vi "Teleop (Christian Colglazier's conflicted copy 2013-02-10).vi"(10 "Match Info":T1={"Autonomous Elapsed Seconds"=0.0, "TeleOp Elapsed Seconds"=0.0, "Disabled Elapsed Seconds"=0.0, "Visited Autonomous"=FALSE, "Visited TeleOp"=FALSE, "Visited Disabled"=FALSE, "Autonomous Settings"={"Autonomous Style"=enum."Independent", "VI Refnum"=refnum}}, 11 "Call Context":T2) -> ()   [LabVIEW 2012]
doc: "This VI is called for each TeleOp packet received from the DS where the robot is not disabled. It is often used to read from the joysticks and update I/O or to update setpoints for timed control loops. It should complete and return within 20 milliseconds or it may miss DS packets."
uses:
  <vilib>/Rock Robotics/WPI/DriverStation/WPI_DriverStationDerivedRobotMode.ctl
  <vilib>/Rock Robotics/WPI/DriverStation/WPI_DriverStationMatch Info.ctl
  Robot Global Data.vi
  <vilib>/Rock Robotics/WPI/Joystick/WPI_JoystickGetSetRefNum.vi
  <vilib>/Rock Robotics/WPI/RobotDrive/WPI_RobotDriveGetSetRefNum.vi
panel:
  out "Numeric 1":dbl(slide) scale=0.0..100.0
  out "Boolean 2":bool
  out "Boolean 1":bool
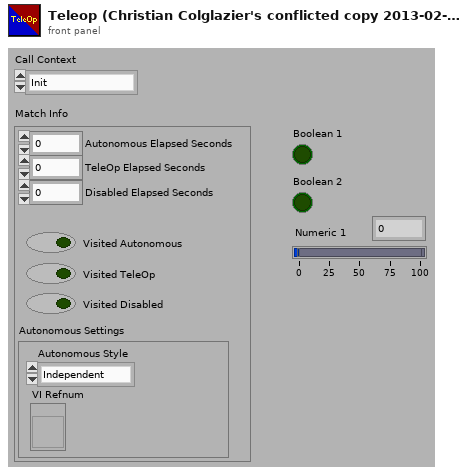
[diagram p1: front panel]
types:
  T1 = typedef "WPI_DriverStationMatch Info.ctl" = cluster{"Autonomous Elapsed Seconds":dbl, "TeleOp Elapsed Seconds":dbl, "Disabled Elapsed Seconds":dbl, "Visited Autonomous":bool, "Visited TeleOp":bool, "Visited Disabled":bool, "Autonomous Settings":cluster{"Autonomous Style":enum16{"Iterative", "Independent"}, "VI Refnum":refnum<vi>}}
  T2 = typedef "WPI_DriverStationDerivedRobotMode.ctl" = enum16{"Init", "Execute", "Stop"}
  T3 = typedef "WPI_RobotDriveDevRef.ctl" = cluster{"DevStatus":errorcluster, "Motors[]":T4[], "Square Inputs":bool, "Max Output":dbl, "Isochronous":bool}
  T4 = typedef "WPI_MotorControlDeviceRef.ctl" = cluster{"DeviceStatus":errorcluster, "Type":enum16{"PWM", "CAN"}, "PWM":cluster{"Digital Module":T5, "PWM Channel":T6, "DeadBand":T7}, "CAN":cluster{"Device Number":u8, "Control Mode":T8, "Semaphore":T9, "Max Vout":dbl}, "Invert":bool, "TransformRef":T10, "InvTransformRef":T10}
  T5 = typedef "FPGA_TypedefDigitalModule.ctl" = enum16{"Digital Module 1", "Digital Module 2"}
  T6 = typedef "FPGA_DIOPWMChannel.ctl" = enum8{"PWM 1", "PWM 2", "PWM 3", "PWM 4", "PWM 5", "PWM 6", "PWM 7", "PWM 8", "PWM 9", "PWM 10", "Invalid"}
  T7 = typedef "WPI_PWMDeadband.ctl" = cluster{"Name":string, "maxPositivePwm":i32, "minPositivePwm":i32, "centerPwm":i32, "maxNegativePwm":i32, "minNegativePwm":i32, "angularRange":u16}
  T8 = typedef "WPI_CANJaguar_ControlMode.ctl" = enum8{"Percent VBus", "Current", "Speed", "Position", "Voltage"}
  T9 = typedef "Semaphore RefNum" = refnum<k1>
  T10 = typedef "WPI_PWMTransform_ConPane.ctl" = refnum<vi>
  T11 = typedef "WPI_JoystickDevRef.ctl" = cluster{"Device":T12}
  T12 = typedef "WPI_JoystickDeviceEnum.ctl" = enum16{"USB 1", "USB 2", "USB 3", "USB 4", "Kinect 1", "Kinect 2"}
  T13 = typedef "WPI_JoystickButtonState.ctl" = cluster{"Button 1":bool, "Button 2":bool, "Button 3":bool, "Button 4":bool, "Button 5":bool, "Button 6":bool, "Button 7":bool, "Button 8":bool, "Button 9":bool, "Button 10":bool, "Button 11":bool, "Button 12":bool}
  T14 = cluster{"axis 1 (x)":dbl, "axis 2 (y)":dbl, "axis 3 (throttle)":dbl, "axis 4":dbl, "axis 5":dbl, "axis 6":dbl}
  T15 = typedef "WPI_AccelerometerDevRef.ctl" = cluster{"DevStatus":errorcluster, "Analog Module":T16, "Analog Channel":T17, "Scaling":T18}
  T16 = typedef "FPGA_TypedefAnalogModule.ctl" = enum16{"Analog Module 1", "Analog Module 2"}
  T17 = typedef "FPGA_AIChannel.ctl" = enum8{"AI 1", "AI 2", "AI 3", "AI 4", "AI 5", "AI 6", "AI 7", "AI 8", "Invalid"}
  T18 = typedef "WPI_AccelerometerScaling.ctl" = cluster{"Gain (VoltsPerG)":dbl, "Center Voltage":dbl}
  T19 = typedef "WPI_GyroDevRef.ctl" = cluster{"DevStatus":errorcluster, "Analog Module":T16, "Analog Channel":T17, "Offset":dbl, "Gain (VoltsPerDegree/Second)":dbl}
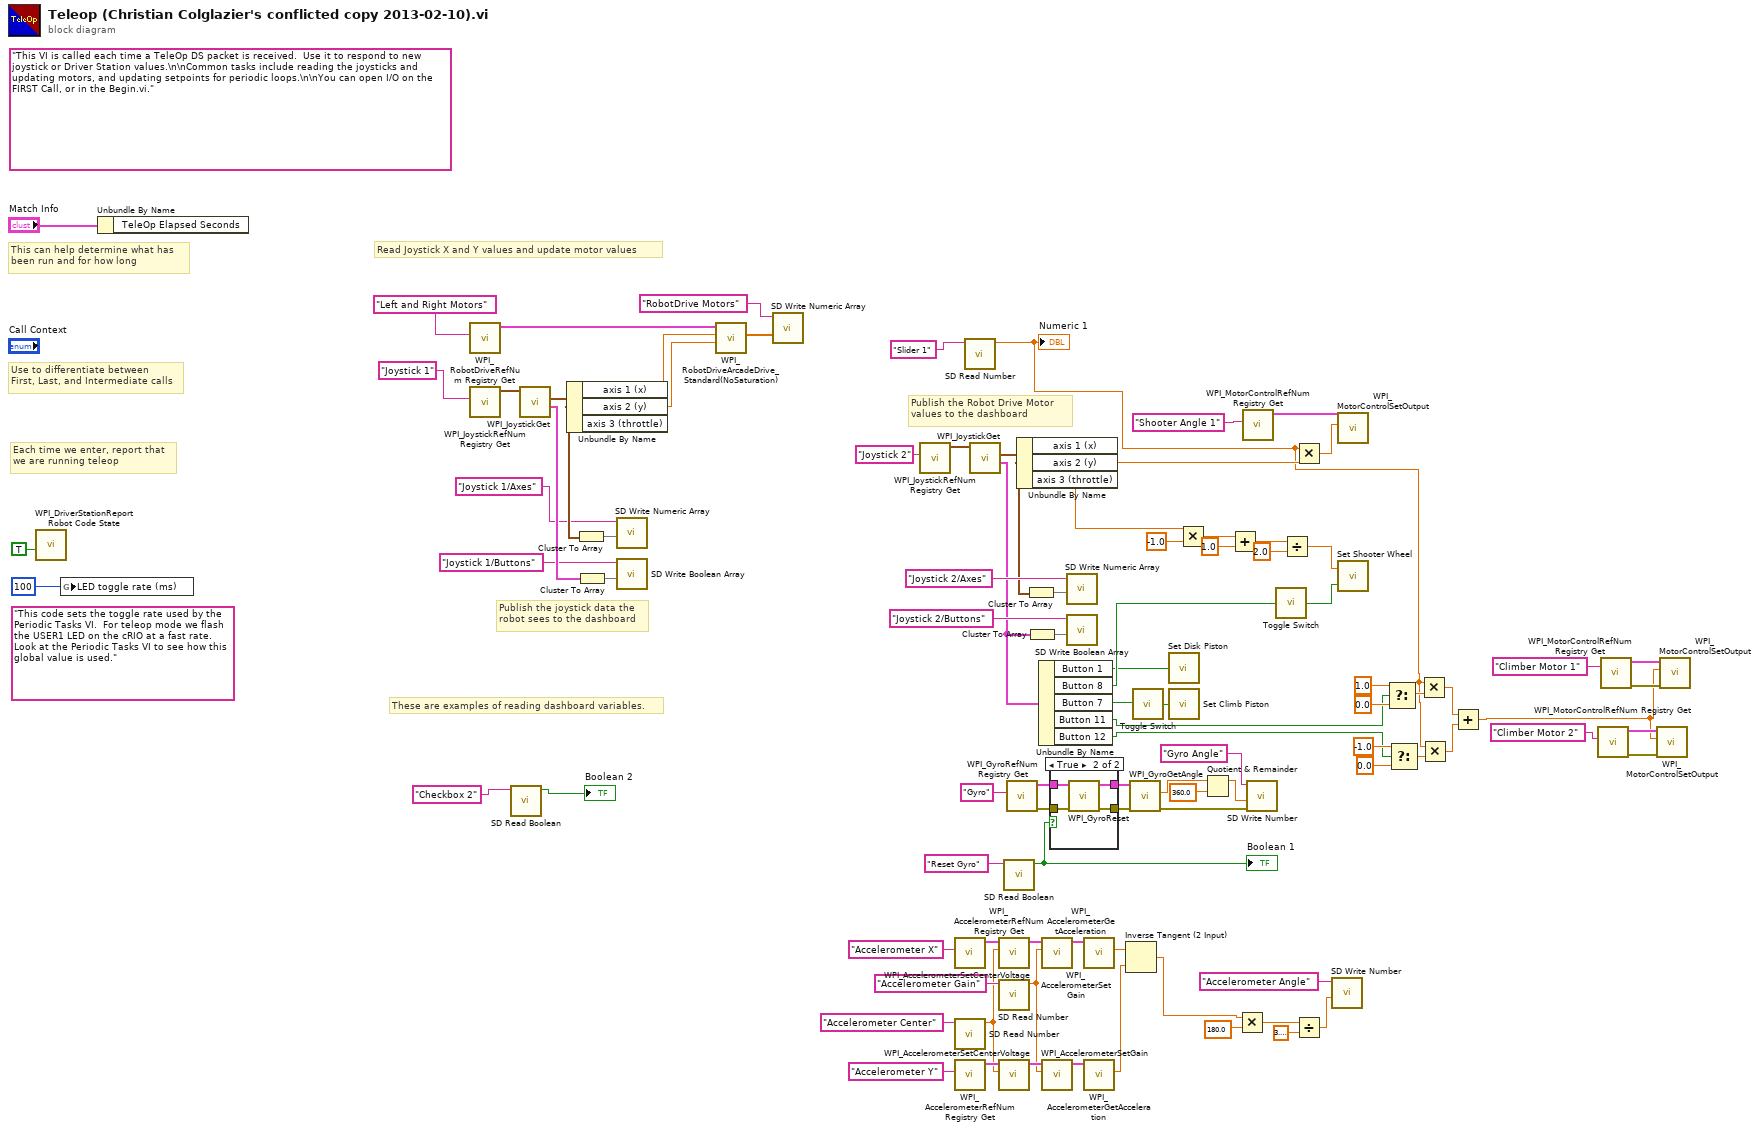
[diagram p0: block diagram]
diagram:
  (unwired) "This code sets the toggle rate used by the Periodic Tasks VI.  For teleop mode we flash the USER1 LED on the cRIO at a fast rate.  Look at the Periodic Tasks VI to see how this global value is used."
  (unwired) "This VI is called each time a TeleOp DS packet is received.  Use it to respond to new joystick or Driver Station values.\n\nCommon tasks include reading the joysticks and updating motors, and updating setpoints for periodic loops.\n\nYou can open I/O on the FIRST Call, or in the Begin.vi."
  # "These are examples of reading dashboard variables."
  # "Publish the Robot Drive Motor\nvalues to the dashboard"
  # "Publish the joystick data the\nrobot sees to the dashboard"
  # "Each time we enter, report that\nwe are running teleop"
  # "Use to differentiate between\nFirst, Last, and Intermediate calls"
  # "This can help determine what has\nbeen run and for how long"
  # "Read Joystick X and Y values and update motor values"
  n1 = call <vilib>:"WPI_DriverStationReport Robot Code State.vi"("TeleOp"=TRUE ("Autonomous")) -> ()  [unwired: 10 in, 1 out]
  n2 = global write "Robot Global Data.vi" "LED toggle rate (ms)"(u32 100 ("LED ms toggle rate")) -> ()
  n3 = Unbundle By Name("Match Info") -> ()  [unwired: 1 out]
  n4 = call <vilib>:"WPI_RobotDriveRefNum Registry Get.vi"("refnum name"="Left and Right Motors") -> ("RobotDriveDevRef"=w92:T3)  [unwired: 1 in, 9 out]
  n5 = call <vilib>:"WPI_JoystickRefNum Registry Get.vi"("refnum name"="Joystick 1") -> ("JoystickDevRef"=w88:T11)  [unwired: 1 in, 9 out]
  n6 = call <vilib>:"SD Read Boolean.vi"("Name"="Checkbox 2" ("refnum name")) -> ("Boolean"=→"Boolean 2":bool)  [unwired: 8 in, 2 out]
  n7 = call <vilib>:"WPI_JoystickGet.vi"("JoystickDevRef"=w88) -> ("Buttons"=w85:T13, "Axes"=w82:T14)  [unwired: 1 in, 4 out]
  n8 = Unbundle By Name(w82) -> ("axis 1 (x)"=w91:dbl, "axis 2 (y)"=w90:dbl)  [unwired: 1 out]
  n9 = Cluster To Array(cluster=w82) -> (array=w81:dbl[])
  n10 = Cluster To Array(cluster=w85) -> (array=w84:bool[])
  n11 = call <vilib>:"SD Write Numeric Array.vi"("Numeric Array"=w81, "Name"="Joystick 1/Axes") -> ()  [unwired: 8 in, 2 out]
  n12 = call <vilib>:"SD Write Boolean Array.vi"("Boolean Array"=w84, "Name"="Joystick 1/Buttons") -> ()  [unwired: 8 in, 2 out]
  n13 = call <vilib>:"WPI_RobotDriveArcadeDrive_Standard(NoSaturation).vi"("Y axis value"=w90, "X axis value"=w91, "RobotDriveDevRef"=w92) -> ("Motor Values"=w78:dbl[])  [unwired: 1 in, 7 out]
  n14 = call <vilib>:"SD Write Numeric Array.vi"("Numeric Array"=w78, "Name"="RobotDrive Motors") -> ()  [unwired: 8 in, 2 out]
  n15 = call <vilib>:"WPI_JoystickRefNum Registry Get.vi"("refnum name"="Joystick 2") -> ("JoystickDevRef"=w68:T11)  [unwired: 1 in, 9 out]
  n16 = call <vilib>:"WPI_AccelerometerRefNum Registry Get.vi"("refnum name"="Accelerometer X") -> ("AccelerometerDevRef"=w26:T15)  [unwired: 9 in, 1 out]
  n17 = call <vilib>:"SD Read Number.vi"("Name"="Accelerometer Center" ("refnum name")) -> ("Numeric"=w21:dbl)  [unwired: 8 in, 2 out]
  n18 = call <vilib>:"WPI_AccelerometerRefNum Registry Get.vi"("refnum name"="Accelerometer Y") -> ("AccelerometerDevRef"=w25:T15)  [unwired: 9 in, 1 out]
  n19 = call <vilib>:"SD Read Number.vi"("Name"="Slider 1" ("refnum name")) -> ("Numeric"=w6:dbl)  [unwired: 8 in, 2 out]
  "Numeric 1" <- w6
  n20 = call <vilib>:"WPI_JoystickGet.vi"("JoystickDevRef"=w68) -> ("Buttons"=w64:T13, "Axes"=w71:T14)  [unwired: 1 in, 4 out]
  n21 = call <vilib>:"WPI_AccelerometerSetCenterVoltage.vi"("Center Voltage"=w21, "AccelerometerDevRef"=w26) -> ("AccelerometerDevRef"=w36:T15)  [unwired: 1 in, 8 out]
  n22 = call <vilib>:"SD Read Number.vi"("Name"="Accelerometer Gain" ("refnum name")) -> ("Numeric"=w22:dbl)  [unwired: 8 in, 2 out]
  n23 = call <vilib>:"WPI_AccelerometerSetCenterVoltage.vi"("Center Voltage"=w21, "AccelerometerDevRef"=w25) -> ("AccelerometerDevRef"=w37:T15)  [unwired: 1 in, 8 out]
  n24 = call <vilib>:"SD Read Boolean.vi"("Name"="Reset Gyro" ("refnum name")) -> ("Boolean"=w46:bool)  [unwired: 8 in, 2 out]
  "Boolean 1" <- w46
  n25 = call <vilib>:"WPI_GyroRefNum Registry Get.vi"("refnum name"="Gyro") -> ("error out"=w41:errorcluster, "GyroDevRef"=w42:T19)  [unwired: 9 in]
  n26 = Unbundle By Name(w71) -> ("axis 2 (y)"=w63:dbl, "axis 3 (throttle)"=w57:dbl)  [unwired: 1 out]
  n27 = Cluster To Array(cluster=w71) -> (array=w72:dbl[])
  n28 = Cluster To Array(cluster=w64) -> (array=w69:bool[])
  n29 = Unbundle By Name(w64) -> ("Button 1"=w52:bool, "Button 8"=w61:bool, "Button 7"=w54:bool, "Button 11"=w14:bool, "Button 12"=w11:bool)
  n30 = call <vilib>:"WPI_AccelerometerSetGain.vi"("Gain (VoltsPerG)"=w22, "AccelerometerDevRef"=w36) -> ("AccelerometerDevRef"=w35:T15)  [unwired: 1 in, 8 out]
  n31 = call <vilib>:"WPI_AccelerometerSetGain.vi"("Gain (VoltsPerG)"=w22, "AccelerometerDevRef"=w37) -> ("AccelerometerDevRef"=w38:T15)  [unwired: 1 in, 8 out]
  n32 = case shown="True" w46 {
    tunnel: w42 -> [w96 w100]
    tunnel: w41 -> [w95 w99]
    tunnel: [w96 w98] -> w40
    tunnel: [w95 w97] -> w39
    frame False {
    }
    frame True {
      n33 = call <vilib>:"WPI_GyroReset.vi"("error in (no error)"=w99, "GyroDevRef"=w100) -> ("error out"=w97:errorcluster, "GyroDevRef"=w98:T19)  [unwired: 8 in]
    }
  }
  n34 = call <vilib>:"SD Write Numeric Array.vi"("Numeric Array"=w72, "Name"="Joystick 2/Axes") -> ()  [unwired: 8 in, 2 out]
  n35 = call <vilib>:"SD Write Boolean Array.vi"("Boolean Array"=w69, "Name"="Joystick 2/Buttons") -> ()  [unwired: 8 in, 2 out]
  n36 = call <vilib>:"WPI_AccelerometerGetAcceleration.vi"("AccelerometerDevRef"=w35) -> ("Acceleration"=w30:dbl)  [unwired: 1 in, 9 out]
  n37 = call <vilib>:"WPI_AccelerometerGetAcceleration.vi"("AccelerometerDevRef"=w38) -> ("Acceleration"=w29:dbl)  [unwired: 1 in, 9 out]
  n38 = Inverse Tangent (2 Input)(1:w29, 2:w30) -> (0:w31:dbl)
  n39 = call <vilib>:"WPI_GyroGetAngle.vi"("error in (no error)"=w39, "GyroDevRef"=w40) -> ("error out"=w48:errorcluster, "Angle"=w44:dbl)  [unwired: 6 in, 2 out]
  n40 = call "Toggle Switch.vi"("OK Button"=w54) -> ("Boolean 2"=w53:bool)
  n41 = call "Set Disk Piston.vi"("Boolean"=w52) -> ()
  n42 = call "Set Climb Piston.vi"("Boolean"=w53) -> ()
  n43 = Multiply(x=w57, y=-1.0) -> (x*y=w56:dbl)
  n44 = Quotient & Remainder(x=w44, y=360.0) -> (x-y*floor(x/y)=w43:dbl)  [unwired: 1 out]
  n45 = Add(x=w56, y=1.0) -> (x+y=w59:dbl)
  n46 = Multiply(x=w31, y=180.0) -> (x*y=w33:dbl)
  n47 = call <vilib>:"WPI_MotorControlRefNum Registry Get.vi"("refnum name"="Shooter Angle 1") -> ("MotorControlDevRef"=w65:T4)  [unwired: 9 in, 1 out]
  n48 = call <vilib>:"SD Write Number.vi"("error in"=w48, "Numeric"=w43, "Name"="Gyro Angle") -> ()  [unwired: 7 in, 2 out]
  n49 = call "Toggle Switch.vi"("OK Button"=w61) -> ("Boolean 2"=w51:bool)
  n50 = Divide(x=w59, y=2.0) -> (x/y=w50:dbl)
  n51 = Multiply(x=w6, y=w63) -> (x*y=w62:dbl)
  n52 = Divide(x=w33, y=3.141592653589793) -> (x/y=w20:dbl)
  n53 = call <vilib>:"SD Write Number.vi"("Numeric"=w20, "Name"="Accelerometer Angle") -> ()  [unwired: 8 in, 2 out]
  n54 = call <vilib>:"WPI_MotorControlSetOutput.vi"("Output"=w62, "MotorControlDevRef"=w65) -> ()  [unwired: 7 in, 3 out]
  n55 = call "Set Shooter Wheel.vi"("Reverse"=w51, "Motor Speed"=w50) -> ()  [unwired: 2 in]
  n56 = Select(t=1.0, s=w14, f=0.0) -> (s? t:f=w9:dbl)
  n57 = Select(t=-1.0, s=w11, f=0.0) -> (s? t:f=w10:dbl)
  n58 = Multiply(x=w6, y=w9) -> (x*y=w7:dbl)
  n59 = Multiply(x=w6, y=w10) -> (x*y=w8:dbl)
  n60 = Add(x=w7, y=w8) -> (x+y=w1:dbl)
  n61 = call <vilib>:"WPI_MotorControlRefNum Registry Get.vi"("refnum name"="Climber Motor 2") -> ("error out"=w3:errorcluster, "MotorControlDevRef"=w2:T4)  [unwired: 9 in]
  n62 = call <vilib>:"WPI_MotorControlRefNum Registry Get.vi"("refnum name"="Climber Motor 1") -> ("error out"=w5:errorcluster, "MotorControlDevRef"=w4:T4)  [unwired: 9 in]
  n63 = call <vilib>:"WPI_MotorControlSetOutput.vi"("error in (no error)"=w3, "Output"=w1, "MotorControlDevRef"=w2) -> ()  [unwired: 6 in, 3 out]
  n64 = call <vilib>:"WPI_MotorControlSetOutput.vi"("error in (no error)"=w5, "Output"=w1, "MotorControlDevRef"=w4) -> ()  [unwired: 6 in, 3 out]
